vi "Cache-FindToExport.vi"(7 "Idx":i32, 8 "error in":errorcluster) -> (0 "error out":errorcluster, 1 "ProductComponent":T1[](array[typedef]), 2 "Results":T2[](array[typedef]))   [LabVIEW 2016]
doc: "Go to DB->WriteStationValues action\nReturn boolean flag to show if data was saved to DB successfully\n\nWabco 2017 All right reserved\nAuthor: maciej.szupienko@wabco-auto.com"
uses:
  Cache.TestSteps.Fglb.ResultData.ctl
  Database/ProdaNG/Controls/ProdaNG.ProcessResult.ctl
  Database/ProdaNG/Controls/ProdaNG.ProcessStepResult.ctl
  Database/ProdaNG/Controls/ProdaNG.TestStepResult.ctl
  Database/ProdaNG/Controls/ProdaNG.TestValueResult.ctl
  Database/ProdaNG/Controls/ProdaNG.ProductComponent.ctl
  Cache.Action.ctl
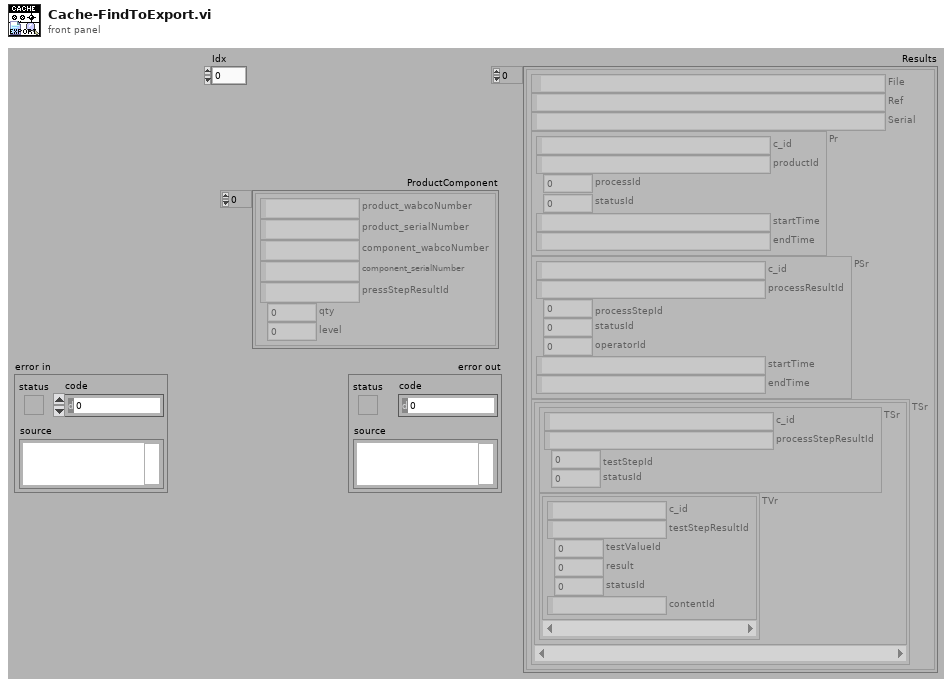
[diagram p1: front panel]
types:
  T1 = typedef "ProdaNG.ProductComponent.ctl" = cluster{"product_wabcoNumber":string, "product_serialNumber":string, "component_wabcoNumber":string, "component_serialNumber":string, "pressStepResultId":string, "qty":i32, "level":i32}
  T2 = typedef "Cache.TestSteps.Fglb.ResultData.ctl" = cluster{"File":path, "Ref":string, "Serial":string, "Pr":T3, "PSr":T4, "TSr":cluster{"TSr":T5, "TVr":T6[]}[]}
  T3 = typedef "ProdaNG.ProcessResult.ctl" = cluster{"c_id":string, "productId":string, "processId":i32, "statusId":i32, "startTime":string, "endTime":string}
  T4 = typedef "ProdaNG.ProcessStepResult.ctl" = cluster{"c_id":string, "processResultId":string, "processStepId":i32, "statusId":i32, "operatorId":i32, "startTime":string, "endTime":string}
  T5 = typedef "ProdaNG.TestStepResult.ctl" = cluster{"c_id":string, "processStepResultId":string, "testStepId":i32, "statusId":i32}
  T6 = typedef "ProdaNG.TestValueResult.ctl" = cluster{"c_id":string, "testStepResultId":string, "testValueId":i32, "result":dbl, "statusId":i32, "contentId":string}
  T7 = typedef "Cache.Action.ctl" = enum32{"idle", "constructor", "destructor", "--- Cache ---", "Find", "FindToExport", "Move", "Delete"}
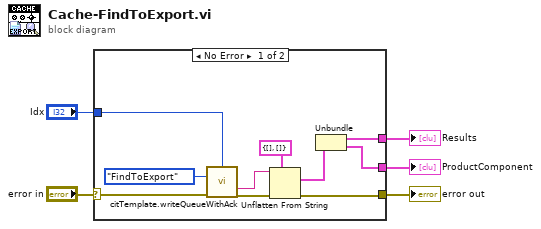
[diagram p0: block diagram]
diagram:
  n1 = case shown="No Error" "error in" {
    selector: "error in" -> [w6 _]
    tunnel: "Idx" -> [w15 _]
    tunnel: [w11 _] -> w4
    tunnel: [w8 _] -> w2
    tunnel: [w10 _] -> w1
    frame No Error {
      n2 = call "citTemplate.writeQueueWithAck.vi"("instance (0)"=w15, "event in"=Cache.Action."FindToExport" ("Action"), "error in (no error)"=w6) -> ("notification data"=w13:string, "error out"=w14:errorcluster)  [unwired: 10 in, 1 out]
      n3 = Unflatten From String(type=cluster{"Results":T2[], "ProductComponent":T1[]} {"Results"=[], "ProductComponent"=[]} ("output cluster"), binary string=w13, error in (no error)=w14) -> (value=w12:cluster{"Results":T2[], "ProductComponent":T1[]}, error out=w11:errorcluster)  [unwired: 2 in, 1 out]
      n4 = Unbundle(w12) -> ("Results"=w8:T2[], "ProductComponent"=w10:T1[])
    }
    frame Error {
    }
  }
  "error out" <- w4
  "Results" <- w2
  "ProductComponent" <- w1
